vi "TranslateLEDUI.vi"(8 "error in (no error)":errorcluster, 11 "GEA2 Reference In":refnum<k24>) -> (0 "error out":errorcluster, 1 "JL_Buttons.ctlJL_LEDs 2":T2, 2 "Tab Control":T1(ring), 3 "GEA2 Reference Out":refnum<k24>, 5 "Convert raw data":string[](array[string]), 7 "LED's Out 0-79":bool[](array[boolean]))   [LabVIEW 2016]
uses:
  Tools/Laundry/JL Dryer Tool/JL Dryer Tool Support/JL_LEDs/JL_LEDs.ctl
  Q:/Common/DLLs/GEA3/GeaCommunication.dll
  Common/DLLs/GEA3/GeaCommunication.dll
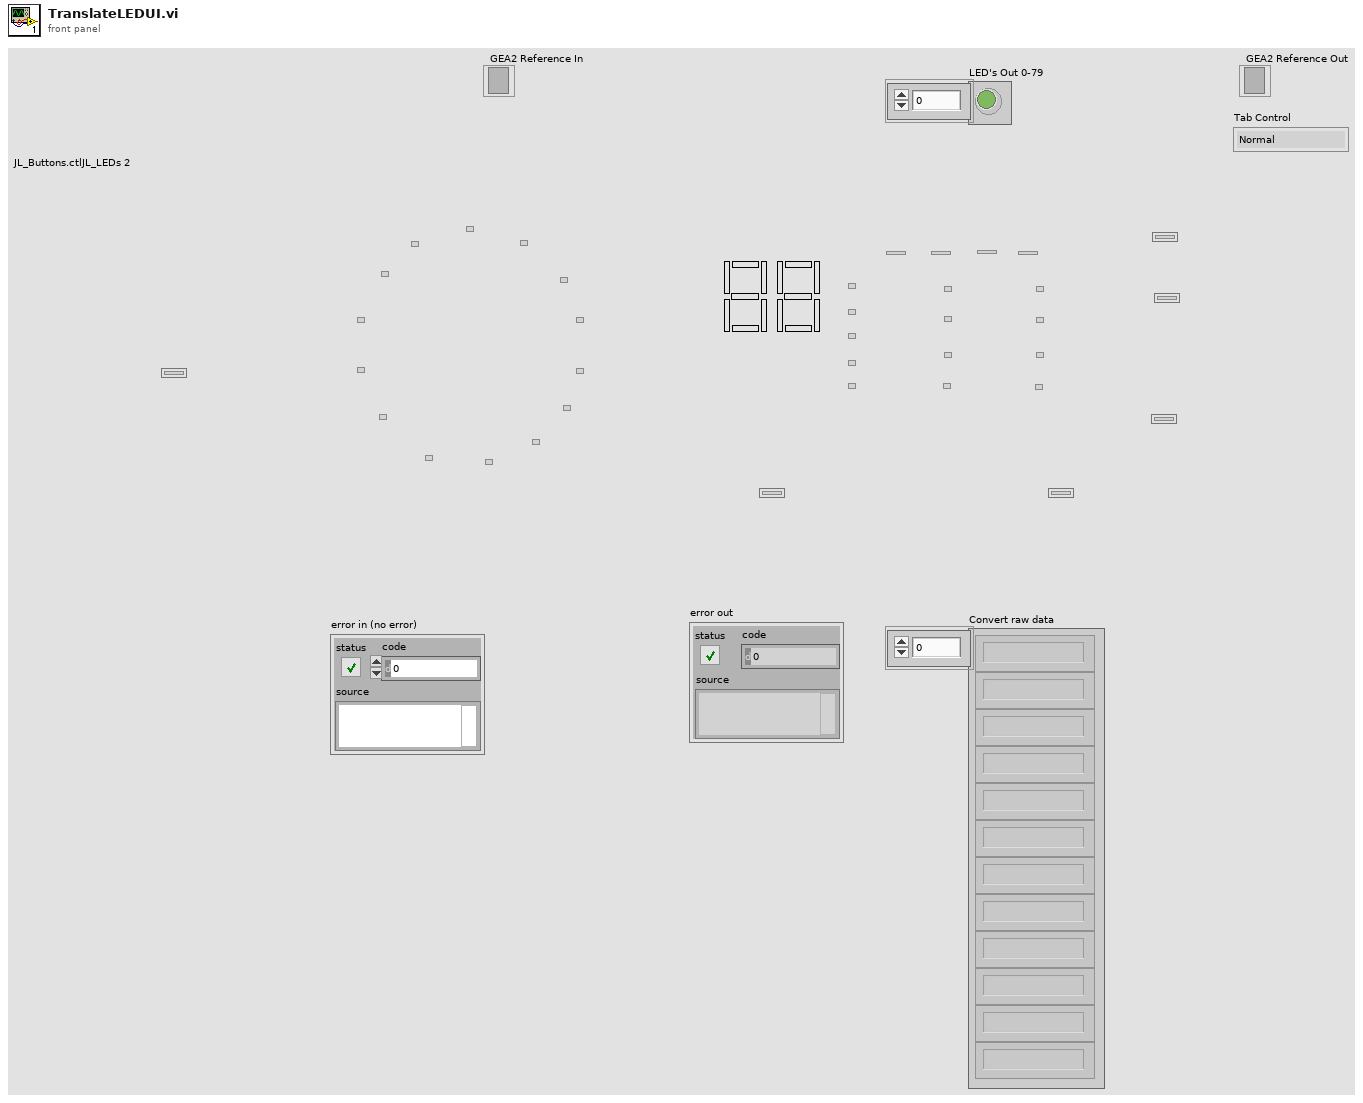
[diagram p1: front panel]
types:
  T1 = enum32{"Normal", "Pause ", "Lock", "Sensing", "Lint Filter"}
  T2 = typedef "JL_LEDs.ctl" = cluster{"Z102 - Start":bool, "Z301 - Encoder 0":bool, "Z302- Encoder 13":bool, "Z303 - Encoder 12":bool, "Z304 - Encoder 11":bool, "Z305 - Encoder 10":bool, "Z306 - Encoder 09":bool, "Z307 - Encoder 08":bool, "Z308- Encoder 07":bool, "Z309 - Encoder 06":bool, "Z310 - Encoder 05":bool, "Z311 - Encoder 04":bool, "Z312 - Encoder 03":bool, "Z313 - Encoder 02":bool, "Z314 - Encoder 01":bool, "Z136 - Pause":bool, "Z137 - Pause":bool, "Z138 - Lock Controls":bool, "Z139 - Lock Controls":bool, "Z140 - Lock Controls":bool, "Z326 - Sensing 1":bool, "Z331 -Sensing 2":bool, "Z353 - Sensing 3":bool, "Delay":bool, "Drying":bool, "Cooling":bool, "Done":bool, "Z101 - Hot":bool, "Z368 - Default Time 4":bool, "Z369 - Default Time 3":bool, "Z372 -Default Time 2":bool, "Z373 - Default Time 1":bool, "Z375 - Default Time 0":bool, "Z383 - More Dry":bool, "Z370 - Dry":bool, "Z388 - Less Dry":bool, "Z391 - Damp":bool, "Z384 - High":bool, "Z385 - Medium":bool, "Z388 - Extra Low":bool, "Z376 - No Heat":bool, "Z351 - Damp Alert":bool, "Z361 - Extended Tumble":bool, "Z358 - eDry":bool, "Z348 -My Cycle":bool, "Z349 - Delay Dry":bool, "Z327 - Clean Lint Filter 1":bool, "Z330 - Clean Lint Filter 2":bool, "Z342 - Clean Lint Filter 3":bool, "Z179 - Pause":bool, "Z109":bool, "Z110":bool, "Z123":bool, "Z124":bool, "Z140":bool, "Unused0":bool, "Unused1":bool, "Unused2":bool, "Unused3":bool, "Channel_Off":bool, "Channel_Cycle_Unmapped":bool, "Z319 - SSD1:G":bool, "Z317 - SSD1:A":bool, "Z318 - SSD1:B":bool, "Z323 - SSD1:F":bool, "Z321 - SSD1:D":bool, "Z320 - SSD1:C":bool, "Z322 - SSD1:E":bool, "Z335 - SSD2:G":bool, "Z333 - SSD2:A":bool, "Z334 - SSD2:B":bool, "Z338 - SSD2:F":bool, "Z336 - SSD2:D":bool, "Z345 - SSD2:C":bool, "Z337 - SSD2:E":bool}
  T3 = typedef "UI_LEDs.ctl" = cluster{"Z301 - Encoder 0":bool, "Z302 - Encoder 13":bool, "Z303 - Encoder 12":bool, "Z304 - Encoder 11":bool, "Z305 - Encoder 10":bool, "Z306 - Encoder 09":bool, "Z307 - Encoder 08":bool, "Z308 - Encoder 07":bool, "Z309 - Encoder 06":bool, "Z310 - Encoder 05":bool, "Z311 - Encoder 04":bool, "Z312 - Encoder 03":bool, "Z313 - Encoder 02":bool, "Z314 - Encoder 01":bool, "Z315 - Unpopulated":bool, "Z316 - Unpopulated":bool, "Z317 - SSD1:A":bool, "Z318 - SSD1:B":bool, "Z319 - SSD1:G":bool, "Z320 - SSD1:C":bool, "Z321 - SSD1:D":bool, "Z322 - SSD1:E":bool, "Z323 - SSD1:F":bool, "Z324 - Pause 1":bool, "Z325 - Control Lock 1":bool, "Z326 - Sensing 1":bool, "Z327 - Clean Lint Filter 1":bool, "Z328 - Extra Status 1":bool, "Z329 - Extra Status 2":bool, "Z330 - Clean Lint Filter 2":bool, "Z331 -Sensing 2":bool, "Z332 - Unpopulated":bool, "Z333 - SSD2:A":bool, "Z334 - SSD2:B":bool, "Z335 - SSD2:G":bool, "Z345 - SSD2:C":bool, "Z336 - SSD2:D":bool, "Z337 - SSD2:E":bool, "Z338 - SSD2:F":bool, "Z339 - Pause 3":bool, "Z340 - Control Lock 3":bool, "Z353 - Sensing 3":bool, "Z342 - Clean Lint Filter 3":bool, "Z344 - Extra Status 3":bool, "Z346 - Extra Status 4":bool, "Z341 - Pause 2":bool, "Z343 - Control Lock 2":bool, "Z347 - Unpopulated":bool, "Z348 -My Cycle":bool, "Z349 - Delay Dry":bool, "Z350 - Volume":bool, "Z351 - Damp Alert":bool, "Z352 - Bar 1":bool, "Z354 - Bar 2":bool, "Z355 - Bar 3":bool, "Z356 - Bar 4":bool, "Z357 - Bar 5":bool, "Z358 - eDry":bool, "Z359 - Time Increment":bool, "Z360 - Time Decrement":bool, "Z361 - Extended Tumble":bool, "Z362 - Unpopulated":bool, "Z363 - Unpopulated":bool, "Z364 - Unpopulated":bool, "Z365 - Status 1":bool, "Z366 - Status 3":bool, "Z367 - Default Time 5":bool, "Z368 - Default Time 4":bool, "Z369 - Default Time 3":bool, "Z370 - Dry":bool, "Z371 - Status 2":bool, "Z372 -Default Time 2":bool, "Z373 - Default Time 1":bool, "Z374 - Unpopulated":bool, "Z375 - Default Time 0":bool, "Z376 - No Heat":bool, "Z377 - Unpopulated":bool, "Z378 - Unpopulated":bool, "Z379 - Unpopulated":bool, "Z380 - Unpopulated":bool, "Z381 - Status 4":bool, "Z382 - Status 6":bool, "Z383 - More Dry":bool, "Z384 - High":bool, "Z385 - Medium":bool, "Z386 -Low":bool, "Z387 - Status 5":bool, "Z388 - Less Dry":bool, "Z388 - Extra Low":bool, "Z390 - Unpopulated":bool, "Z391 - Damp":bool, "Z392 - Unpopulated":bool, "Z393 - Unpopulated":bool, "Z394 - Unpopulated":bool, "Z395 - Unpopulated":bool, "Z396 - Unpopulated":bool, "Z101 - unpop?":bool, "Z102 - Start/Pause":bool, "OFF - OFF":bool, "MAX - MAX":bool}
  T4 = typedef "SB_LEDs.ctl" = cluster{"Z101 - Start/Pause":bool, "Z - unpop?":bool, "Z103 - Encoder 0":bool, "Z104 - Encoder 13":bool, "Z105 - Encoder 12":bool, "Z106 - Encoder 11":bool, "Z107 - Encoder 10":bool, "Z108 - Encoder 09":bool, "Z109 - Encoder 08":bool, "Z110 - Encoder 07":bool, "Z111 - Encoder 06":bool, "Z112 - Encoder 05":bool, "Z113 - Encoder 04":bool, "Z114 - Encoder 03":bool, "Z115 - Encoder 02":bool, "Z116 - Encoder 01":bool, "Z117 - Bar 1":bool, "Z118 - Bar 2":bool, "Z119 - Bar 3":bool, "Z120 - Bar 4":bool, "Z121 - Bar 5":bool, "Z122 - SSD1:A":bool, "Z123 - SSD1:B":bool, "Z124 - SSD1:C":bool, "Z125 - SSD1:D":bool, "Z126 - SSD1:E":bool, "Z127 - SSD1:F":bool, "Z128 - SSD1:G":bool, "Z129 - SSD2:A":bool, "Z130 - SSD2:B":bool, "Z131 - SSD2:C":bool, "Z132 - SSD2:D":bool, "Z133 - SSD2:E":bool, "Z134 - SSD2:F":bool, "Z135 - SSD2:G":bool, "Z136 - Pause 2":bool, "Z137 - Pause 3":bool, "Z138 - Control Lock 1":bool, "Z139 - Control Lock 2":bool, "Z140 - Control Lock 3":bool, "Z142 - Sensing 1":bool, "Z142 -Sensing 2":bool, "Z143 - Sensing 3":bool, "Z144 - Extra Status 1":bool, "Z145 - Extra Status 2":bool, "Z146 - Extra Status 3":bool, "Z147 - Extra Status 4":bool, "Z148 - Status 1":bool, "Z149 - Status 2":bool, "Z150 - Status 3":bool, "Z151 - Status 4":bool, "Z152 - Status 5":bool, "Z153 - Status 6":bool, "Z154 - Default Time 5":bool, "Z155 - Default Time 4":bool, "Z153 - Default Time 3":bool, "Z157 -Default Time 2":bool, "Z158 - Default Time 1":bool, "Z159 - Default Time 0":bool, "Z160 - More Dry":bool, "Z161 - Dry":bool, "Z162 - Less Dry":bool, "Z163 - Damp":bool, "Z164 - High":bool, "Z165 - Medium":bool, "Z166 - Extra Low":bool, "Z167 - No Heat":bool, "Z168 - Volume":bool, "Z169 - Damp Alert":bool, "Z170 - Extended Tumble":bool, "Z171 - Time Decrement":bool, "Z172 - Time Increment":bool, "Z173 - eDry":bool, "Z174 -My Cycle":bool, "Z175 - Delay Dry":bool, "Z176 - Clean Lint Filter 1":bool, "Z177 - Clean Lint Filter 2":bool, "Z178 - Clean Lint Filter 3":bool, "Z179 - Pause 1":bool, "OFF - OFF":bool, "MAX - MAX":bool, "Z165B -Low":bool}
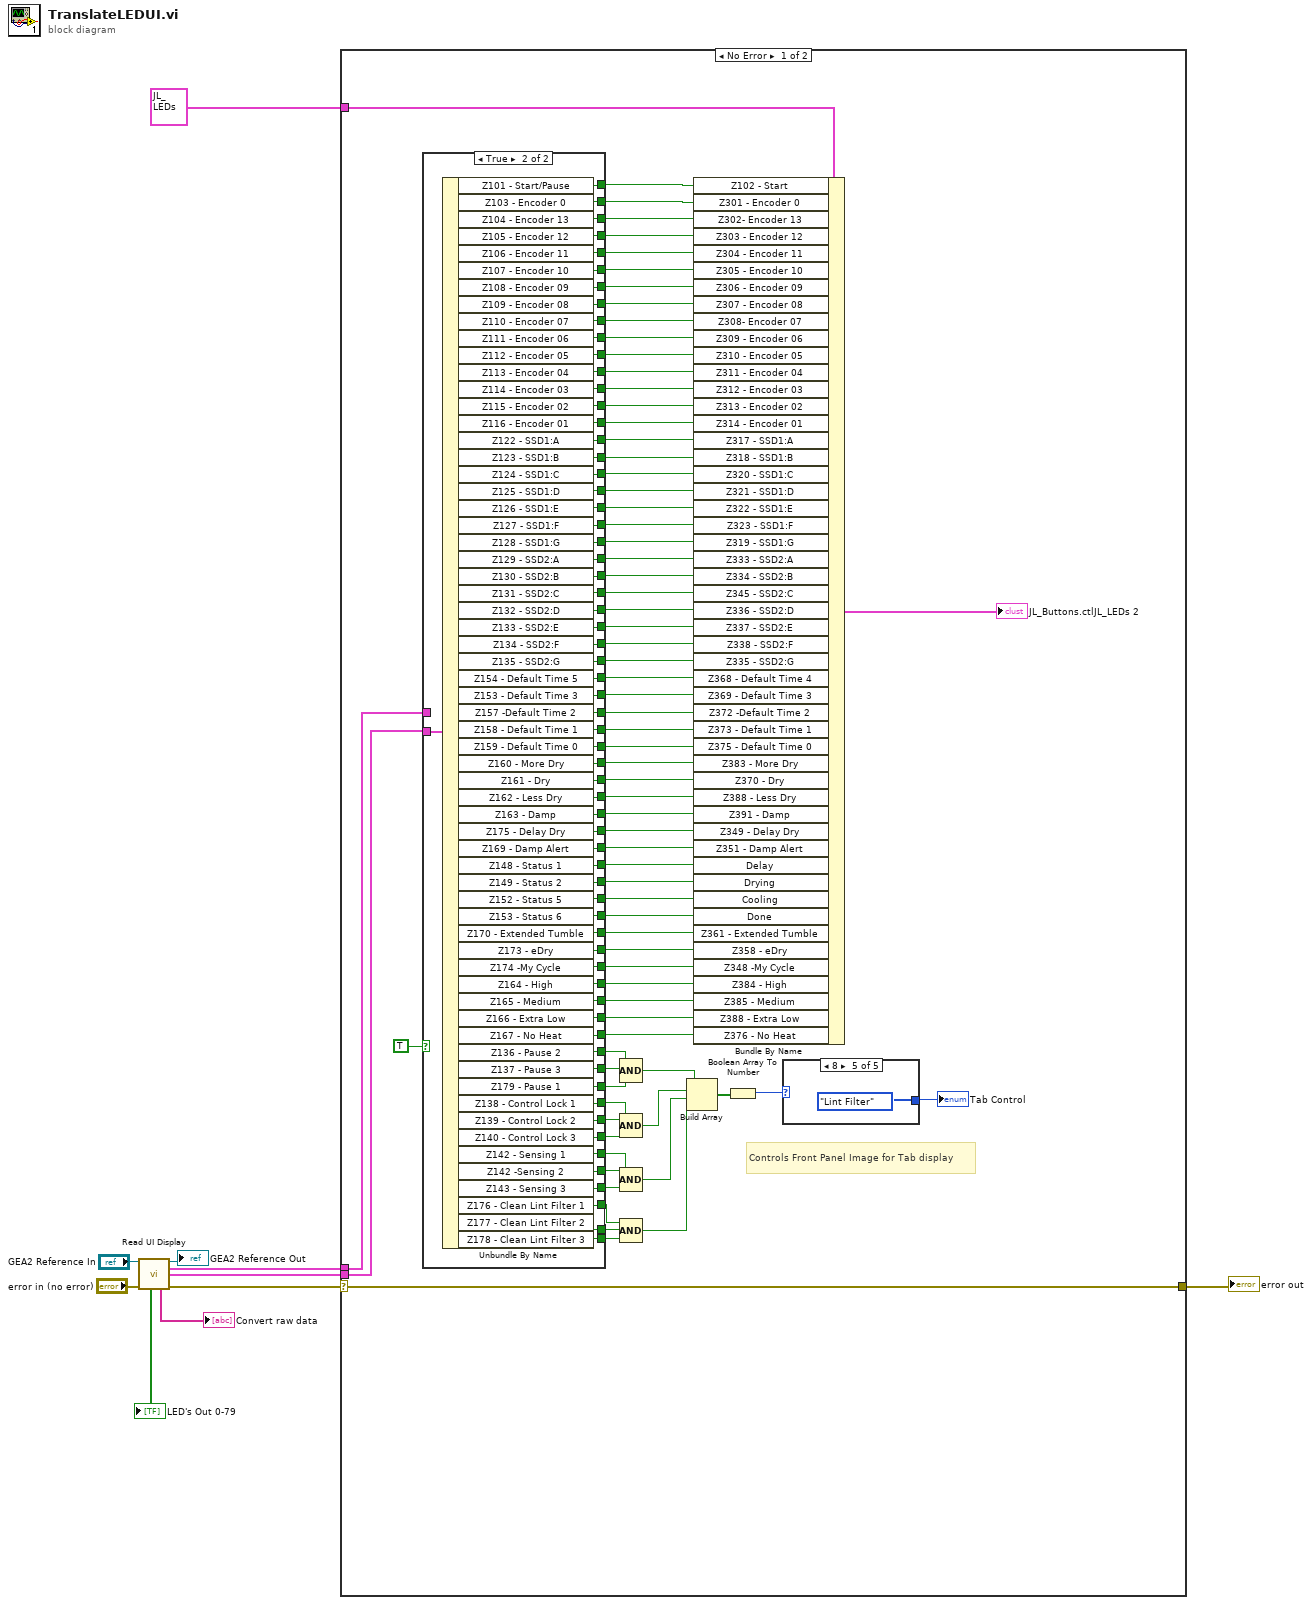
[diagram p0: block diagram]
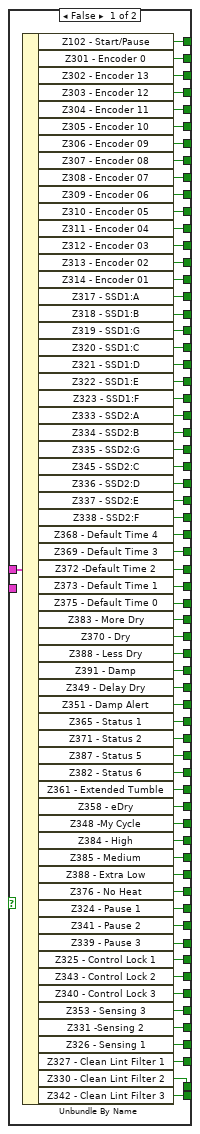
[diagram p2: hidden frame]
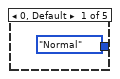
[diagram p3: hidden frame]
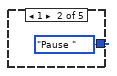
[diagram p4: hidden frame]
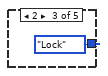
[diagram p5: hidden frame]
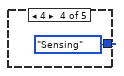
[diagram p6: hidden frame]
diagram:
  n1 = call "Read UI Display.vi"("GEA2 Reference In"="GEA2 Reference In", "Error In"="error in (no error)") -> ("GEA2 Reference Out"=→"GEA2 Reference Out":refnum<k24>, "Justice League UI"=w7:T3, "Justice League SB"=w3:T4, "LED's Out 0-79"=→"LED's Out 0-79":bool[], "Convert raw data"=→"Convert raw data":string[], "Error Out"=w8:errorcluster)  [unwired: 8 in]
  n2 = case shown="No Error" w8 {
    selector: w8 -> [w17 _]
    tunnel: [w17 _] -> w10
    tunnel: w7 -> [w18 _]
    tunnel: T2 {"Z102 - Start"=FALSE, "Z301 - Encoder 0"=FALSE, "Z302- Encoder 13"=FALSE, "Z303 - Encoder 12"=FALSE, "Z304 - Encoder 11"=FALSE, "Z305 - Encoder 10"=FALSE, "Z306 - Encoder 09"=FALSE, "Z307 - Encoder 08"=FALSE, "Z308- Encoder 07"=FALSE, "Z309 - Encoder 06"=FALSE, "Z310 - Encoder 05"=FALSE, "Z311 - Encoder 04"=FALSE, "Z312 - Encoder 03"=FALSE, "Z313 - Encoder 02"=FALSE, "Z314 - Encoder 01"=FALSE, "Z136 - Pause"=FALSE, "Z137 - Pause"=FALSE, "Z138 - Lock Controls"=FALSE, "Z139 - Lock Controls"=FALSE, "Z140 - Lock Controls"=FALSE, "Z326 - Sensing 1"=FALSE, "Z331 -Sensing 2"=FALSE, "Z353 - Sensing 3"=FALSE, "Delay"=FALSE, "Drying"=FALSE, "Cooling"=FALSE, "Done"=FALSE, "Z101 - Hot"=FALSE, "Z368 - Default Time 4"=FALSE, "Z369 - Default Time 3"=FALSE, "Z372 -Default Time 2"=FALSE, "Z373 - Default Time 1"=FALSE, "Z375 - Default Time 0"=FALSE, "Z383 - More Dry"=FALSE, "Z370 - Dry"=FALSE, "Z388 - Less Dry"=FALSE, "Z391 - Damp"=FALSE, "Z384 - High"=FALSE, "Z385 - Medium"=FALSE, "Z388 - Extra Low"=FALSE, "Z376 - No Heat"=FALSE, "Z351 - Damp Alert"=FALSE, "Z361 - Extended Tumble"=FALSE, "Z358 - eDry"=FALSE, "Z348 -My Cycle"=FALSE, "Z349 - Delay Dry"=FALSE, "Z327 - Clean Lint Filter 1"=FALSE, "Z330 - Clean Lint Filter 2"=FALSE, "Z342 - Clean Lint Filter 3"=FALSE, "Z179 - Pause"=FALSE, "Z109"=FALSE, "Z110"=FALSE, "Z123"=FALSE, "Z124"=FALSE, "Z140"=FALSE, "Unused0"=FALSE, "Unused1"=FALSE, "Unused2"=FALSE, "Unused3"=FALSE, "Channel_Off"=FALSE, "Channel_Cycle_Unmapped"=FALSE, "Z319 - SSD1:G"=FALSE, "Z317 - SSD1:A"=FALSE, "Z318 - SSD1:B"=FALSE, "Z323 - SSD1:F"=FALSE, "Z321 - SSD1:D"=FALSE, "Z320 - SSD1:C"=FALSE, "Z322 - SSD1:E"=FALSE, "Z335 - SSD2:G"=FALSE, "Z333 - SSD2:A"=FALSE, "Z334 - SSD2:B"=FALSE, "Z338 - SSD2:F"=FALSE, "Z336 - SSD2:D"=FALSE, "Z345 - SSD2:C"=FALSE, "Z337 - SSD2:E"=FALSE} ("JL_Buttons.ctlJL_LEDs 2") -> [w16 _]
    tunnel: w3 -> [w12 _]
    frame No Error {
      # "Controls Front Panel Image for Tab display"
      n3 = case shown="True" TRUE {
        tunnel: [w150 w212] -> w85
        tunnel: [w149 w214] -> w84
        tunnel: [w148 w211] -> w83
        tunnel: [w147 w199] -> w82
        tunnel: [w146 w210] -> w81
        tunnel: [w145 w209] -> w80
        tunnel: [w144 w208] -> w79
        tunnel: [w143 w207] -> w78
        tunnel: [w142 w206] -> w77
        tunnel: [w141 w205] -> w76
        tunnel: [w140 w204] -> w75
        tunnel: [w139 w203] -> w74
        tunnel: [w138 w202] -> w73
        tunnel: [w137 w201] -> w72
        tunnel: [w136 w200] -> w71
        tunnel: [w135 w198] -> w70
        tunnel: [w134 w197] -> w69
        tunnel: [w133 w196] -> w68
        tunnel: [w132 w195] -> w67
        tunnel: [w131 w194] -> w66
        tunnel: [w130 w193] -> w11
        tunnel: [w129 w192] -> w13
        tunnel: [w128 w185] -> w65
        tunnel: [w127 w186] -> w64
        tunnel: [w126 w187] -> w63
        tunnel: [w125 w188] -> w62
        tunnel: [w124 w189] -> w61
        tunnel: [w123 w190] -> w60
        tunnel: [w122 w191] -> w59
        tunnel: [w121 w184] -> w58
        tunnel: [w120 w183] -> w57
        tunnel: [w119 w182] -> w56
        tunnel: [w118 w181] -> w55
        tunnel: [w117 w180] -> w54
        tunnel: [w116 w176] -> w53
        tunnel: [w115 w177] -> w52
        tunnel: [w114 w178] -> w51
        tunnel: [w113 w179] -> w50
        tunnel: [w112 w175] -> w49
        tunnel: [w111 w174] -> w48
        tunnel: [w110 w170] -> w47
        tunnel: [w109 w171] -> w46
        tunnel: [w108 w172] -> w45
        tunnel: [w107 w173] -> w44
        tunnel: [w106 w168] -> w14
        tunnel: [w105 w169] -> w43
        tunnel: [w104 w167] -> w42
        tunnel: [w103 w166] -> w41
        tunnel: [w102 w165] -> w40
        tunnel: [w101 w164] -> w39
        tunnel: [w100 w163] -> w38
        tunnel: [w99 w160] -> w37
        tunnel: [w98 w161] -> w36
        tunnel: [w97 w162] -> w35
        tunnel: [w96 w159] -> w34
        tunnel: [w95 w158] -> w33
        tunnel: [w94 w157] -> w32
        tunnel: [w93 w156] -> w31
        tunnel: [w92 w155] -> w30
        tunnel: [w91 w154] -> w29
        tunnel: [w90 w153] -> w28
        tunnel: [w89 w152] -> w27
        tunnel: [w88 w151] -> w26
        tunnel: w18 -> [w87 _]
        tunnel: w12 -> [_ w213]
        frame False {
          n4 = Unbundle By Name(w87) -> ("Z102 - Start/Pause"=w149:bool, "Z301 - Encoder 0"=w150:bool, "Z302 - Encoder 13"=w148:bool, "Z303 - Encoder 12"=w146:bool, "Z304 - Encoder 11"=w145:bool, "Z305 - Encoder 10"=w144:bool, "Z306 - Encoder 09"=w143:bool, "Z307 - Encoder 08"=w142:bool, "Z308 - Encoder 07"=w141:bool, "Z309 - Encoder 06"=w140:bool, "Z310 - Encoder 05"=w139:bool, "Z311 - Encoder 04"=w138:bool, "Z312 - Encoder 03"=w137:bool, "Z313 - Encoder 02"=w136:bool, "Z314 - Encoder 01"=w147:bool, "Z317 - SSD1:A"=w135:bool, "Z318 - SSD1:B"=w134:bool, "Z319 - SSD1:G"=w133:bool, "Z320 - SSD1:C"=w132:bool, "Z321 - SSD1:D"=w131:bool, "Z322 - SSD1:E"=w130:bool, "Z323 - SSD1:F"=w129:bool, "Z333 - SSD2:A"=w122:bool, "Z334 - SSD2:B"=w123:bool, "Z335 - SSD2:G"=w124:bool, "Z345 - SSD2:C"=w125:bool, "Z336 - SSD2:D"=w126:bool, "Z337 - SSD2:E"=w127:bool, "Z338 - SSD2:F"=w128:bool, "Z368 - Default Time 4"=w121:bool, "Z369 - Default Time 3"=w120:bool, "Z372 -Default Time 2"=w119:bool, "Z373 - Default Time 1"=w118:bool, "Z375 - Default Time 0"=w117:bool, "Z383 - More Dry"=w113:bool, "Z370 - Dry"=w114:bool, "Z388 - Less Dry"=w115:bool, "Z391 - Damp"=w116:bool, "Z349 - Delay Dry"=w112:bool, "Z351 - Damp Alert"=w111:bool, "Z365 - Status 1"=w107:bool, "Z371 - Status 2"=w108:bool, "Z387 - Status 5"=w109:bool, "Z382 - Status 6"=w110:bool, "Z361 - Extended Tumble"=w105:bool, "Z358 - eDry"=w106:bool, "Z348 -My Cycle"=w104:bool, "Z384 - High"=w100:bool, "Z385 - Medium"=w101:bool, "Z388 - Extra Low"=w102:bool, "Z376 - No Heat"=w103:bool, "Z324 - Pause 1"=w99:bool, "Z341 - Pause 2"=w98:bool, "Z339 - Pause 3"=w97:bool, "Z325 - Control Lock 1"=w96:bool, "Z343 - Control Lock 2"=w95:bool, "Z340 - Control Lock 3"=w94:bool, "Z353 - Sensing 3"=w93:bool, "Z331 -Sensing 2"=w92:bool, "Z326 - Sensing 1"=w91:bool, "Z327 - Clean Lint Filter 1"=w90:bool, "Z330 - Clean Lint Filter 2"=w89:bool, "Z342 - Clean Lint Filter 3"=w88:bool)
        }
        frame True {
          n5 = Unbundle By Name(w213) -> ("Z101 - Start/Pause"=w214:bool, "Z103 - Encoder 0"=w212:bool, "Z104 - Encoder 13"=w211:bool, "Z105 - Encoder 12"=w210:bool, "Z106 - Encoder 11"=w209:bool, "Z107 - Encoder 10"=w208:bool, "Z108 - Encoder 09"=w207:bool, "Z109 - Encoder 08"=w206:bool, "Z110 - Encoder 07"=w205:bool, "Z111 - Encoder 06"=w204:bool, "Z112 - Encoder 05"=w203:bool, "Z113 - Encoder 04"=w202:bool, "Z114 - Encoder 03"=w201:bool, "Z115 - Encoder 02"=w200:bool, "Z116 - Encoder 01"=w199:bool, "Z122 - SSD1:A"=w198:bool, "Z123 - SSD1:B"=w197:bool, "Z124 - SSD1:C"=w196:bool, "Z125 - SSD1:D"=w195:bool, "Z126 - SSD1:E"=w194:bool, "Z127 - SSD1:F"=w193:bool, "Z128 - SSD1:G"=w192:bool, "Z129 - SSD2:A"=w191:bool, "Z130 - SSD2:B"=w190:bool, "Z131 - SSD2:C"=w189:bool, "Z132 - SSD2:D"=w188:bool, "Z133 - SSD2:E"=w187:bool, "Z134 - SSD2:F"=w186:bool, "Z135 - SSD2:G"=w185:bool, "Z154 - Default Time 5"=w184:bool, "Z153 - Default Time 3"=w183:bool, "Z157 -Default Time 2"=w182:bool, "Z158 - Default Time 1"=w181:bool, "Z159 - Default Time 0"=w180:bool, "Z160 - More Dry"=w179:bool, "Z161 - Dry"=w178:bool, "Z162 - Less Dry"=w177:bool, "Z163 - Damp"=w176:bool, "Z175 - Delay Dry"=w175:bool, "Z169 - Damp Alert"=w174:bool, "Z148 - Status 1"=w173:bool, "Z149 - Status 2"=w172:bool, "Z152 - Status 5"=w171:bool, "Z153 - Status 6"=w170:bool, "Z170 - Extended Tumble"=w169:bool, "Z173 - eDry"=w168:bool, "Z174 -My Cycle"=w167:bool, "Z164 - High"=w163:bool, "Z165 - Medium"=w164:bool, "Z166 - Extra Low"=w165:bool, "Z167 - No Heat"=w166:bool, "Z136 - Pause 2"=w160:bool, "Z137 - Pause 3"=w161:bool, "Z179 - Pause 1"=w162:bool, "Z138 - Control Lock 1"=w159:bool, "Z139 - Control Lock 2"=w158:bool, "Z140 - Control Lock 3"=w157:bool, "Z142 - Sensing 1"=w156:bool, "Z142 -Sensing 2"=w155:bool, "Z143 - Sensing 3"=w154:bool, "Z176 - Clean Lint Filter 1"=w153:bool, "Z177 - Clean Lint Filter 2"=w152:bool, "Z178 - Clean Lint Filter 3"=w151:bool)
        }
      }
      n6 = Compound Arithmetic op=AND(w37, w36, w35) -> (w23:bool)
      n7 = Compound Arithmetic op=AND(w34, w33, w32) -> (w22:bool)
      n8 = Compound Arithmetic op=AND(w31, w30, w29) -> (w21:bool)
      n9 = Compound Arithmetic op=AND(w28, w27, w26) -> (w19:bool)
      n10 = Build Array(w23, w22, w21, w19) -> (w25:bool[])
      n11 = Bundle By Name(cluster=w16, "Z102 - Start"=w84, "Z301 - Encoder 0"=w85, "Z302- Encoder 13"=w83, "Z303 - Encoder 12"=w81, "Z304 - Encoder 11"=w80, "Z305 - Encoder 10"=w79, "Z306 - Encoder 09"=w78, "Z307 - Encoder 08"=w77, "Z308- Encoder 07"=w76, "Z309 - Encoder 06"=w75, "Z310 - Encoder 05"=w74, "Z311 - Encoder 04"=w73, "Z312 - Encoder 03"=w72, "Z313 - Encoder 02"=w71, "Z314 - Encoder 01"=w82, "Z317 - SSD1:A"=w70, "Z318 - SSD1:B"=w69, "Z320 - SSD1:C"=w68, "Z321 - SSD1:D"=w67, "Z322 - SSD1:E"=w66, "Z323 - SSD1:F"=w11, "Z319 - SSD1:G"=w13, "Z333 - SSD2:A"=w59, "Z334 - SSD2:B"=w60, "Z345 - SSD2:C"=w61, "Z336 - SSD2:D"=w62, "Z337 - SSD2:E"=w63, "Z338 - SSD2:F"=w64, "Z335 - SSD2:G"=w65, "Z368 - Default Time 4"=w58, "Z369 - Default Time 3"=w57, "Z372 -Default Time 2"=w56, "Z373 - Default Time 1"=w55, "Z375 - Default Time 0"=w54, "Z383 - More Dry"=w50, "Z370 - Dry"=w51, "Z388 - Less Dry"=w52, "Z391 - Damp"=w53, "Z349 - Delay Dry"=w49, "Z351 - Damp Alert"=w48, "Delay"=w44, "Drying"=w45, "Cooling"=w46, "Done"=w47, "Z361 - Extended Tumble"=w43, "Z358 - eDry"=w14, "Z348 -My Cycle"=w42, "Z384 - High"=w38, "Z385 - Medium"=w39, "Z388 - Extra Low"=w40, "Z376 - No Heat"=w41) -> (→"JL_Buttons.ctlJL_LEDs 2":T2)
      n12 = Boolean Array To Number(Boolean array=w25) -> (number=w24:u32)
      n13 = case shown="8" w24 {
        tunnel: [T1."Normal" ("Tab Control") T1."Pause " ("Tab Control") T1."Lock" ("Tab Control") T1."Sensing" ("Tab Control") T1."Lint Filter" ("Tab Control")] -> w20
        frame 0, Default {
        }
        frame 1 {
        }
        frame 2 {
        }
        frame 4 {
        }
        frame 8 {
        }
      }
      "Tab Control" <- w20
    }
    frame Error {
    }
  }
  "error out" <- w10
